vi "Launch POLARIS TA Focus.vi"() -> ()   [LabVIEW 2014, in "POLARIS Target Focus Actor.lvlib"]
uses:
  POLARIS Target Focus Actor.lvlib
  POLARIS Target Focus Actor/POLARIS Target Focus Actor.lvclass
  <vilib>/ActorFramework/Actor/Actor.lvclass
panel:
  out "error out":errorcluster
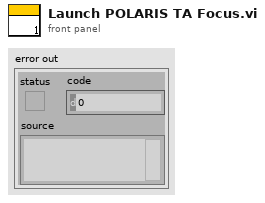
[diagram p1: front panel]
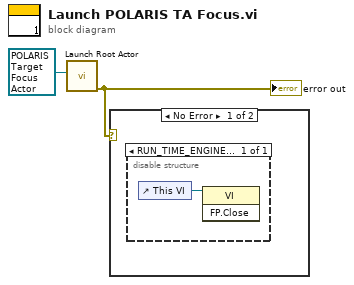
[diagram p0: block diagram]
diagram:
  n1 = call <vilib>:"Launch Root Actor.vi"("Actor"=refnum<class "POLARIS Target Focus Actor.lvclass"> refnum ("POLARIS Target Focus Actor.lvlib:POLARIS Target Focus Actor.lvclass")) -> ("error out"=w1:errorcluster)  [unwired: 9 in, 1 out]
  "error out" <- w1
  n2 = case shown="No Error" w1 {
    frame No Error {
      n3 = disable-structure shown="RUN_TIME_ENGINE==True, Default" {
        frame condition #0 (active) {
          n4 = control-ref of="This VI"() -> (w3:refnum<vi>)
          n5 = invoke class="VI" method="FP.Close"(reference=w3) -> ()  [unwired: 2 in, 3 out]
        }
      }
    }
    frame Error {
    }
  }
